vi "AWS-S3-Transfer-Abort.vi"(0 "AWS-S3-API":refnum<class "AWS-S3-API.lvclass">, 11 "error in":errorcluster) -> (4 "AWS-S3-API out":refnum<class "AWS-S3-API.lvclass">, 15 "error out":errorcluster)   [LabVIEW 2012, in "AWS-S3-API.lvclass"]
uses:
  AWS-S3-API.lvclass
  C:/Users/Jack/repo/aws/AWS-SDK/AWSSDK.dll
  repo/aws/AWS-SDK/AWSSDK.dll
panel:
  # "Inputs"
  # "Outputs"
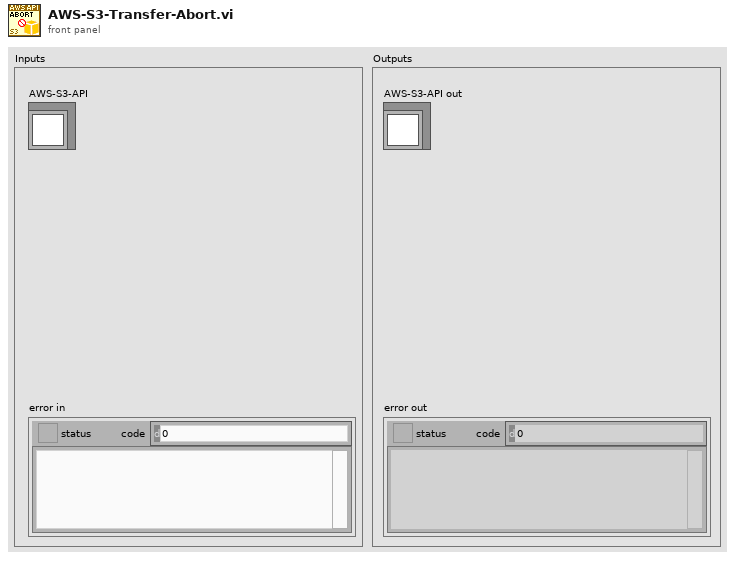
[diagram p1: front panel]
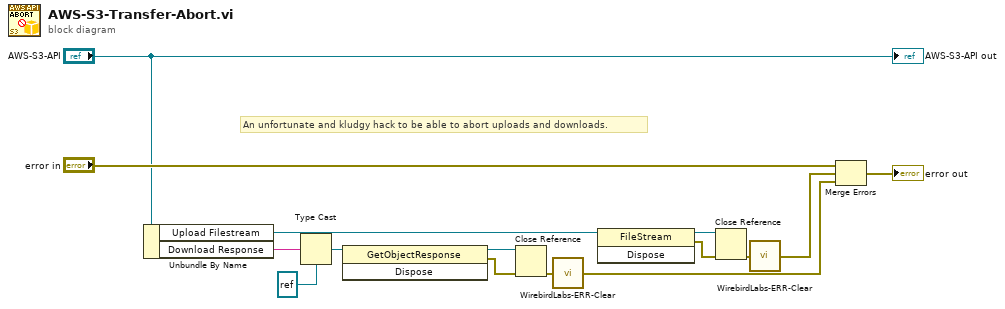
[diagram p0: block diagram]
diagram:
  # "An unfortunate and kludgy hack to be able to abort uploads and downloads."
  n1 = Unbundle By Name("AWS-S3-API") -> ("Upload Filestream"=w4:refnum<k24>, "Download Response"=w3:string)
  n2 = Type Cast(type=refnum<k24> refnum, x=w3) -> (*(type *) &x=w2:refnum<k24>)
  n3 = invoke class="GetObjectResponse" method="Dispose"(reference=w2) -> (reference out=w11:refnum<k24>, error out=w10:errorcluster)  [unwired: 2 in, 1 out]
  n4 = Close Reference(reference=w11, error in (no error)=w10) -> (error out=w9:errorcluster)
  n5 = call "WirebirdLabs-ERR-Clear.vi"("error to snuff"=w9) -> ("no error"=w12:errorcluster)
  n6 = invoke class="FileStream" method="Dispose"(reference=w4) -> (reference out=w8:refnum<k24>, error out=w7:errorcluster)  [unwired: 2 in, 1 out]
  n7 = Close Reference(reference=w8, error in (no error)=w7) -> (error out=w6:errorcluster)
  n8 = call "WirebirdLabs-ERR-Clear.vi"("error to snuff"=w6) -> ("no error"=w13:errorcluster)
  n9 = Merge Errors("error in", w13, w12) -> (→"error out":errorcluster)
  "AWS-S3-API out" <- "AWS-S3-API"
